vi "Assert Message Given Inputs.vi"(6 "Identical Inputs Comparator":refnum<class "Comparator.lvclass">, 7 "Expected Message":string, 8 "error in (no error)":errorcluster, 9 "Call 2":variant, 10 "Call 1":variant, 11 "Comparator Message Test in":refnum<class "Comparator Message Test.lvclass">) -> (0 "error out":errorcluster, 3 "Comparator Message Test out":refnum<class "Comparator Message Test.lvclass">)   [LabVIEW 2020, in "Comparator Message Test.lvclass"]
uses:
  Comparator Message Test.lvclass
  source/Core/Comparator/Comparator.lvclass
  C:/Program Files (x86)/National Instruments/LabVIEW 2020/vi.lib/Astemes/LUnit/Test Case.lvclass
  <vilib>/Astemes/LUnit/Test Case.lvclass/Test Case.ctl
  bb6a28c9-3dc4-4ef9-9c40-faae2425c9ad.vi
  <vilib>/Astemes/LUnit/Append Pass Result.vi
  <vilib>/Astemes/LUnit/Append Fail Result.vi
  <vilib>/Astemes/LUnit/Describe Comparison.vi
  <vilib>/Astemes/LUnit/Compare Variants.vi
  <vilib>/Astemes/LUnit/Variant to string.vi
  Test Doubles/Mock VI Call/Mock VI Call.lvclass
  C:/git/astemes-lmock/source/Core/VI Call/VI Call.lvclass
  <vilib>/Utility/Data Type/Get Type Information.vi
  <vilib>/Utility/LVClass/Get LV Class Name.vi
  Comparator Message Test.lvclass/Comparator Message Test.ctl
  C:/git/astemes-lmock/source/Framework/VI Server VI Call/VI Server VI Call.lvclass
  C:/git/astemes-lmock/tests/Test Doubles/Mock VI Call/Mock VI Call.lvclass
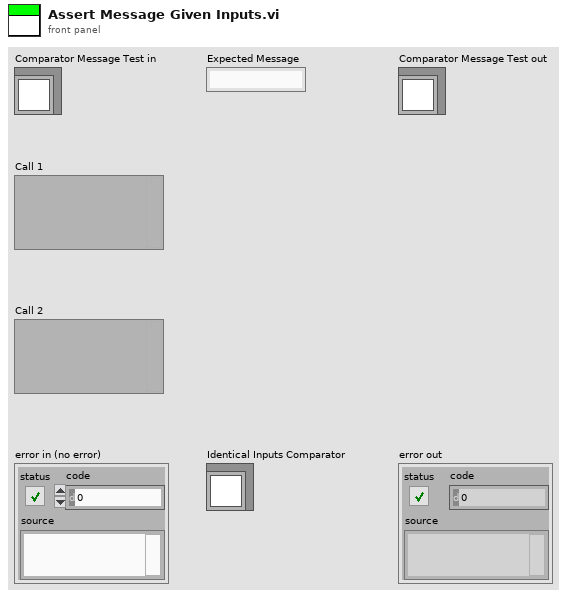
[diagram p1: front panel]
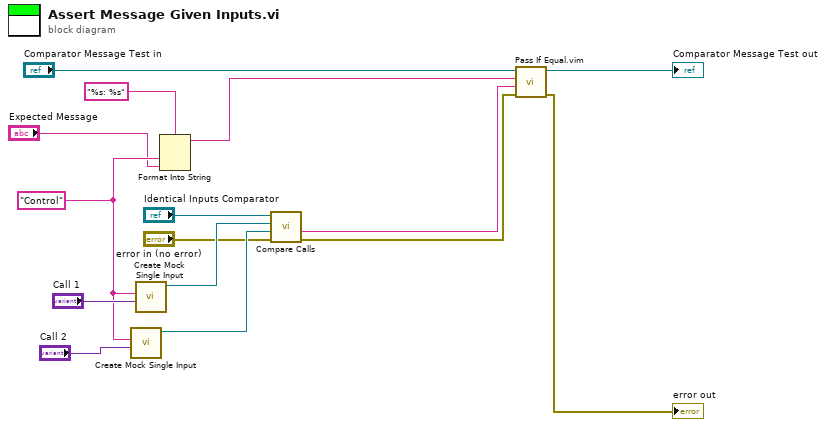
[diagram p0: block diagram]
diagram:
  w3 = "Control" ("Control Label")
  n1 = call "Create Mock Single Input.vi"("Control value"="Call 2", "Control Label"=w3) -> ("Mock VI Call Out"=w11:refnum<class "Mock VI Call.lvclass">)  [unwired: 8 in, 1 out]
  n2 = call "Create Mock Single Input.vi"("Control value"="Call 1", "Control Label"=w3) -> ("Mock VI Call Out"=w10:refnum<class "Mock VI Call.lvclass">)  [unwired: 8 in, 1 out]
  n3 = Format Into String(format string="%s: %s", w3, "Expected Message") -> (resulting string=w1:string)  [unwired: 2 in, 1 out]
  n4 = call-dynamic "Compare Calls.vi"("error in (no error)"="error in (no error)", "VI Call 2"=w11, "VI Call 1"=w10, "Comparator in"="Identical Inputs Comparator") -> ("error out"=w14:errorcluster, "Description"=w15:string)  [unwired: 5 in, 1 out]
  n5 = call "Pass If Equal.vim"("error in (no error)"=w14, "Actual"=w15, "Expected"=w1, "LUnit Test Case In"="Comparator Message Test in") -> ("error out"=→"error out":errorcluster, "LUnit Test Case Out"=→"Comparator Message Test out":refnum<class "Comparator Message Test.lvclass">)  [unwired: 6 in]
